vi "Red Pitaya Manager back.vi"() -> ()   [LabVIEW 2024]
uses:
  Libraries/Red Pitaya/RP Calibration.ctl
  Libraries/Red Pitaya/RP Calibration 4ch.ctl
  Libraries/Red Pitaya/RP Channel Calibration.ctl
  Libraries/Red Pitaya/RP Filter 4ch.ctl
  Libraries/Red Pitaya/RP Channel Filter.ctl
  Libraries/Red Pitaya/RP Calibration 2ch.ctl
  Libraries/Red Pitaya/RP Core/RP Communicator/RP Communicator.lvclass
  Libraries/Red Pitaya/RP Command.ctl
  Libraries/Red Pitaya/RP Config Offsets.ctl
  Libraries/Red Pitaya/RP Status Offsets.ctl
  <vilib>/regexp/Match Regular Expression.xnode
  Libraries/Red Pitaya/Red Pitaya Digitizer/Red Pitaya Digitizer.lvclass
panel:
  in  "Find Red Pitayas":bool
  out "Calibration":T1
  out "output cluster":T1
  in  "Tab Control":enum32{"Manage", "Settings", "Diagnostics"}(tab)
  in  "Frequencies":dbl[](array[numeric])=[0.0, 0.0]
  in  "Out enable":bool[](array[boolean])
  in  "Out gains":dbl[](array[numeric])=[1.0, 1.0]
  in  "Out offsets":i16[](array[numeric])=[0, 0]
  in  "Reset calibration":bool
  out "Waveform Chart":dbl[][](graph)
  in  "Input ranges":bool[](array[boolean])=[FALSE, FALSE, FALSE, FALSE]
  in  "In offsets":i32[](array[numeric])
  in  "In gains":dbl[](array[numeric])
  out "Calibrating":bool
  in  "Write callibration":bool
  in  "Stop calibration":bool
  in  "Start calibration":bool
  out "Starup script":string
  in  "View  startup":bool
  in  "View  bitfiles":bool
  in  "Red Pitayas":i32(listbox)
  out "bit files":string
  in  "bitfile functionality":string[](array[string])=["variable-rate digitizer", "lockin-digitizer", "slow lockin-digitizer", "lockin-digitizer  for 122.88", "fast 4-ch digitizer", "critical current", "slow critical current", "variable rate 4-ch digitizer"]
  in  "Bitfile logic tags 2":u16[](array[numeric])=[152, 159, 164, 169, 157, 154, 155, 158]
  in  "Subnet":string="192.168.1"
  in  "Start address":i32=100
  in  "End address":i32=120
  in  "Bitfile logic tags":u16[](array[numeric])=[101, 102, 109, 113, 159, 157, 152, 158]
  in  "Timeout":i32=100
  out "Bitfile IDs map":map{u16, string}(c390)={152="variable-rate digitizer", 154="critical current", 155="slow critical current", 157="fast 4-ch digitizer", 159="lockin-digitizer", 164="slow lockin-digitizer", 169="lockin-digitizer  for 122.88"}
  out "Addresses":string[](array[string])
  out "Device names":string[](array[string])
  out "Modules":i32[](array[numeric])
  out "DDS modula out":i64[](array[numeric])=[101, 102]
  out "Logic tags out":u16[](array[numeric])=[101, 102]
  in  "error in":errorcluster
  out "error out":errorcluster
  out "standard output":string
  out "standard error":string
  in  "Exit Button":bool
  # "typedef enum {\n    STEM_125_10_v1_0            = 0,\n    STEM_125_14_v1_0            = 1,\n    STEM_125_14_v1_1            = 2,\n    STEM_122_16SDR_v1_0         = 3,\n    STEM_122_16SDR_v1_1         = 4,\n    STEM_125_14_LN_v1_1         = 5,\n    STEM_125_14_Z7020_v1_0      = 6,\n    STEM_125_14_Z7020_LN_v1_1   = 7,\n    STEM_125_14_Z7020_4IN_v1_0  = 8,\n    STEM_125_14_Z7020_4IN_v1_2  = 9,\n    STEM_125_14_Z7020_4IN_v1_3  = 10,\n    STEM_250_12_v1_0            = 11,\n    STEM_250_12_v1_1            = 12,\n    STEM_250_12_v1_2            = 13,\n    STEM_250_12_120             = 14,\n    STEM_250_12_v1_2a           = 15,\n    STEM_250_12_v1_2b           = 16,\n    STEM_125_14_LN_BO_v1_1      = 17,\n    STEM_125_14_LN_CE1_v1_1     = 18,\n    STEM_125_14_LN_CE2_v1_1     = 19\n}  rp_HPeModels_t;"
  # "typedef enum {\n    Z7010 = 0,\n    Z7020 = 1\n}  rp_HPeZynqModels_t;"
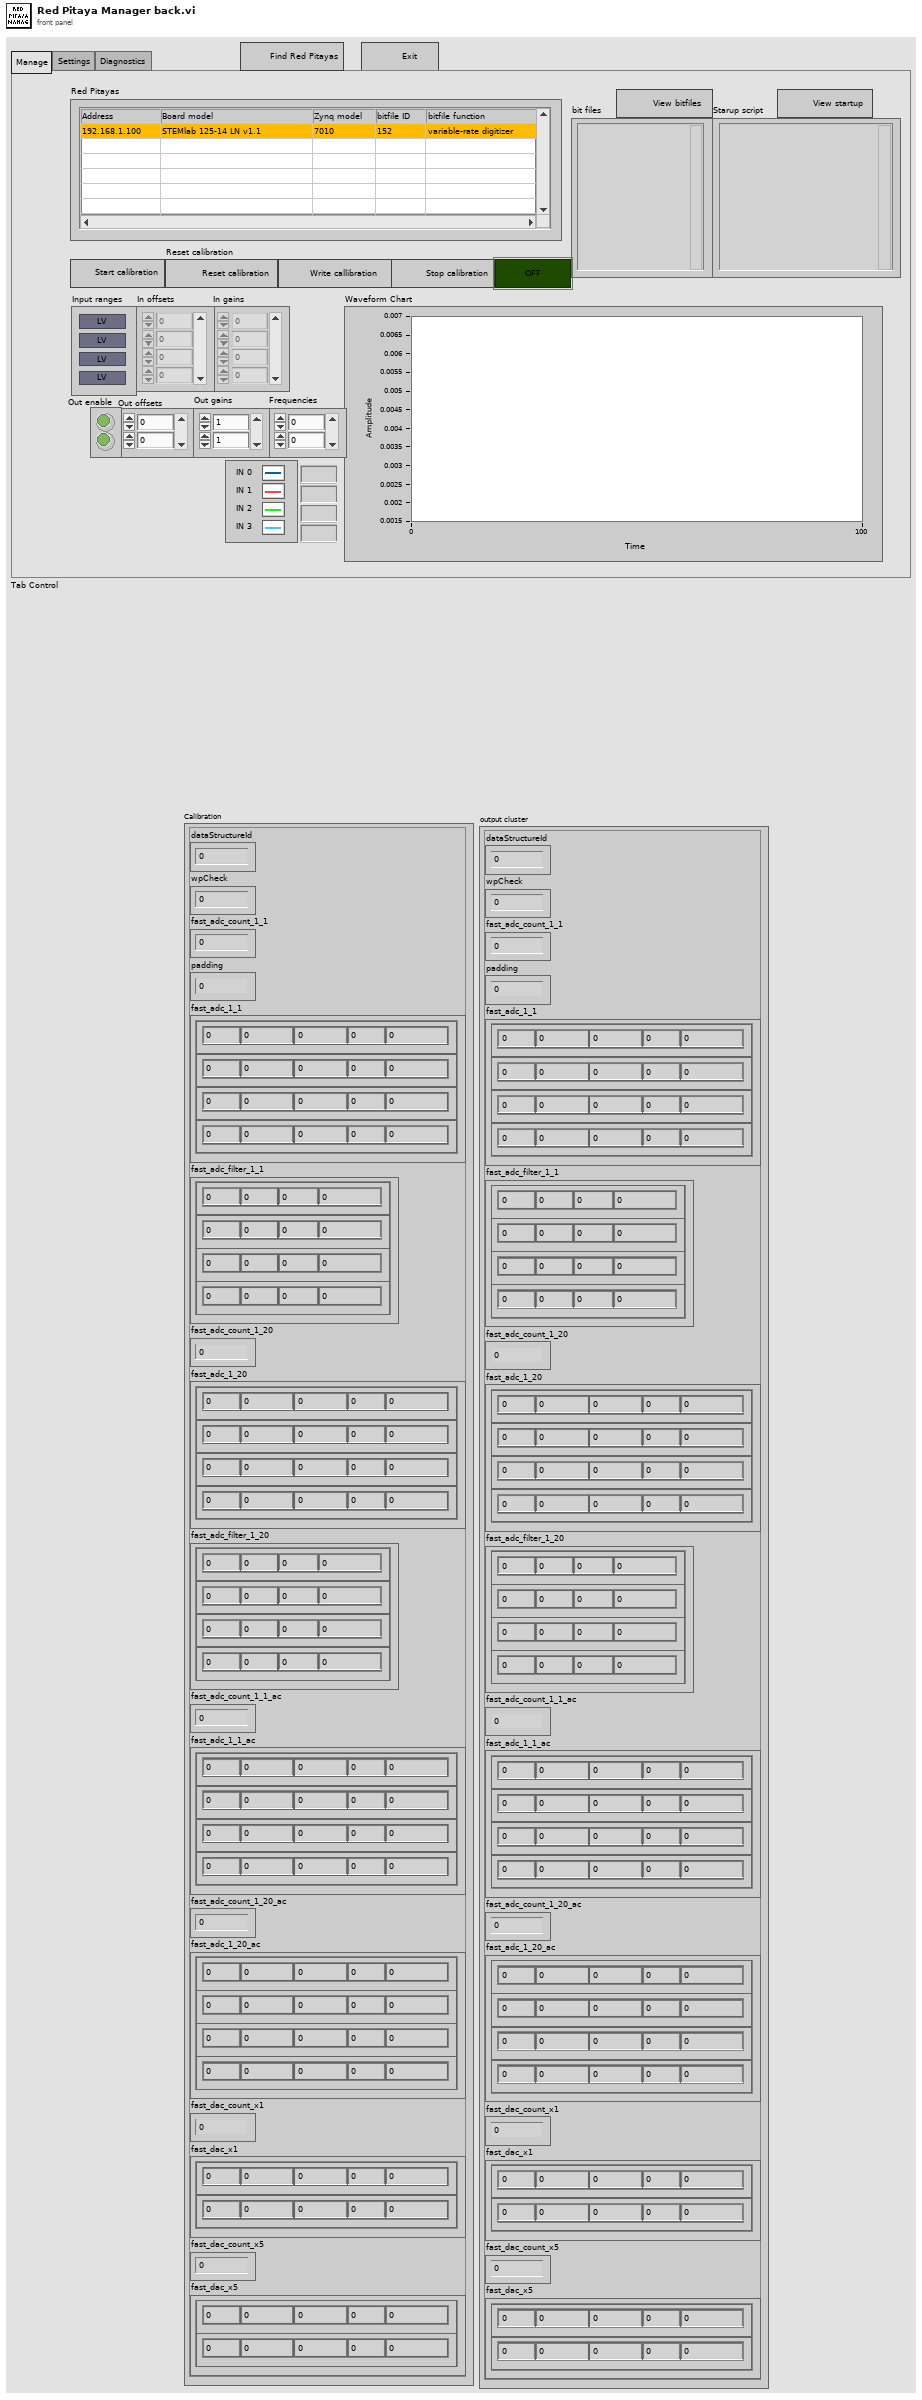
[diagram p1: front panel]
types:
  T1 = typedef "RP Calibration.ctl" = cluster{"dataStructureId":u8, "wpCheck":u8, "fast_adc_count_1_1":u16, "padding":u32, "fast_adc_1_1":T2, "fast_adc_filter_1_1":T4, "fast_adc_count_1_20":u64, "fast_adc_1_20":T2, "fast_adc_filter_1_20":T4, "fast_adc_count_1_1_ac":u64, "fast_adc_1_1_ac":T2, "fast_adc_count_1_20_ac":u64, "fast_adc_1_20_ac":T2, "fast_dac_count_x1":u64, "fast_dac_x1":T6, "fast_dac_count_x5":u64, "fast_dac_x5":T6}
  T2 = typedef "RP Calibration 4ch.ctl" = cluster{"ch_0":T3, "ch_1":T3, "ch_2":T3, "ch_3":T3}
  T3 = typedef "RP Channel Calibration.ctl" = cluster{"baseScale":sgl, "calibValue":u32, "offset":i32, "padding 2":i32, "gainCalc":dbl}
  T4 = typedef "RP Filter 4ch.ctl" = cluster{"ch_0":T5, "ch_1":T5, "ch_2":T5, "ch_3":T5}
  T5 = typedef "RP Channel Filter.ctl" = cluster{"aa":u32, "bb":u32, "pp":u32, "kk":u32}
  T6 = typedef "RP Calibration 2ch.ctl" = cluster{"ch_0":T3, "ch_1":T3}
  T7 = typedef "RP Command.ctl" = enum16{"Reset", "Read IDN", "Stop server", "Get status", "Get temperature", "Connect client", "Arm", "Software trigger", "Get whole buffer", "Get chunk", "System call", "Get config", "Set config", "Recieve data", "Recieve Calibartion", "Transmit data"}
  T8 = typedef "RP Config Offsets.ctl" = u16
  T9 = typedef "RP Status Offsets.ctl" = u16
  T10 = cluster{"fast_dac_x1[0]":T3, "fast_dac_x1[1]":T3}
  T11 = cluster{"fast_adc_1_1[0]":T3, "fast_adc_1_1[1]":T3, "fast_adc_1_1[2]":T3, "fast_adc_1_1[3]":T3}
  T12 = cluster{"fast_adc_1_20[0]":T3, "fast_adc_1_20[1]":T3, "fast_adc_1_20[2]":T3, "fast_adc_1_20[3]":T3}
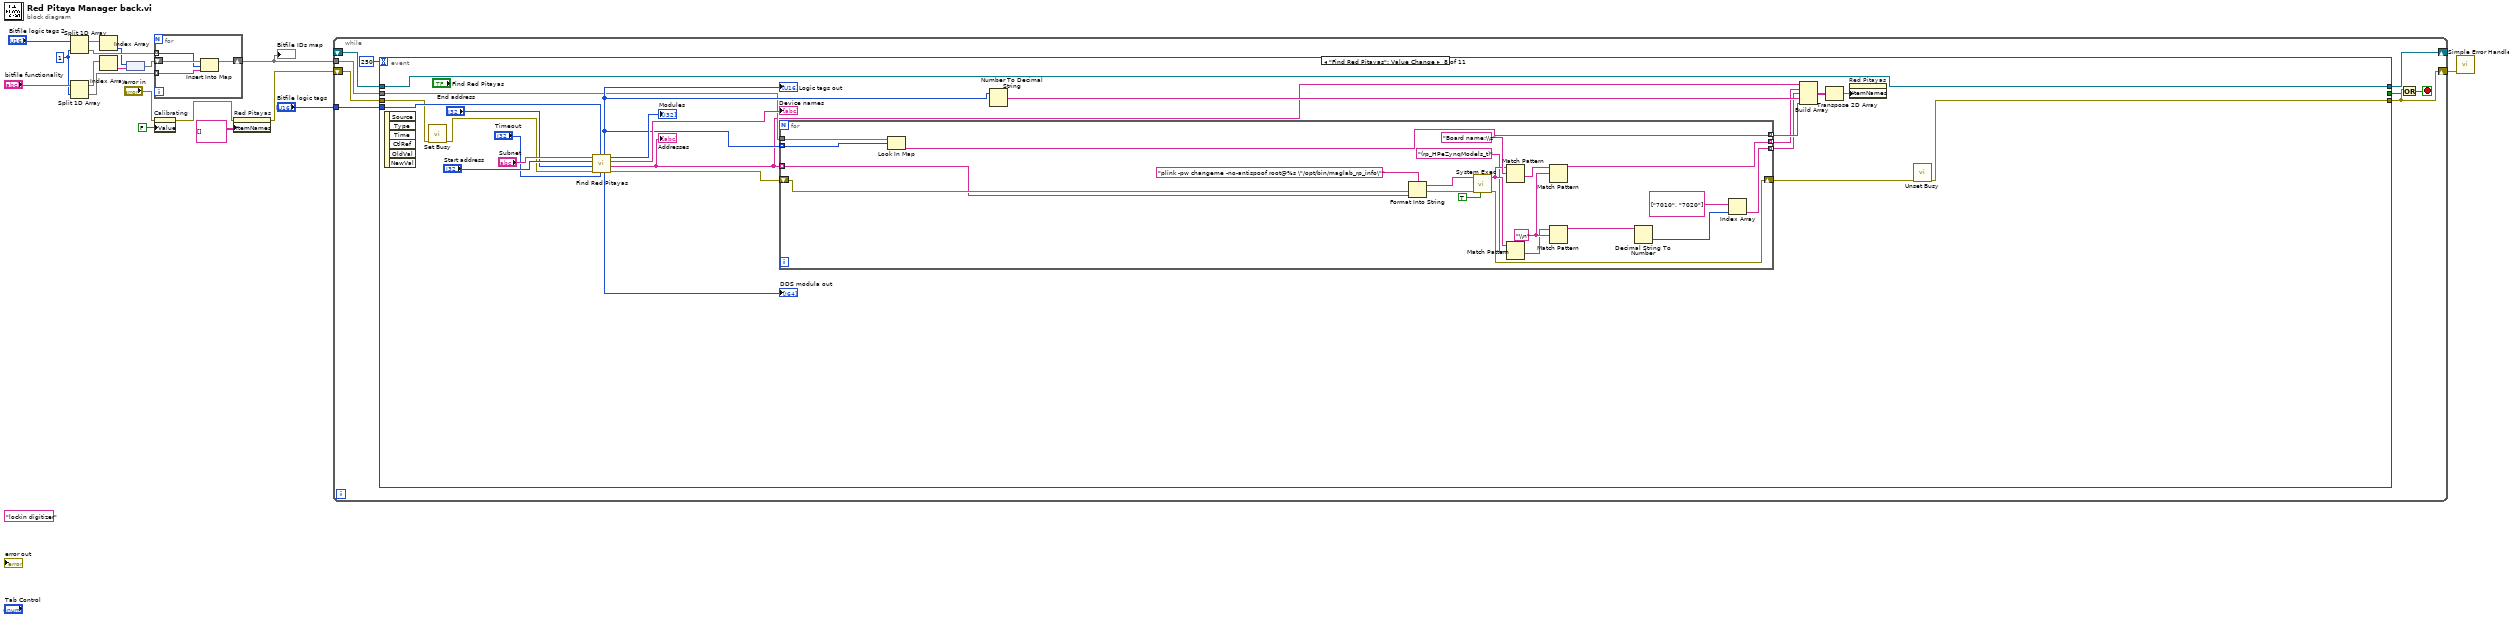
[diagram p0: block diagram]
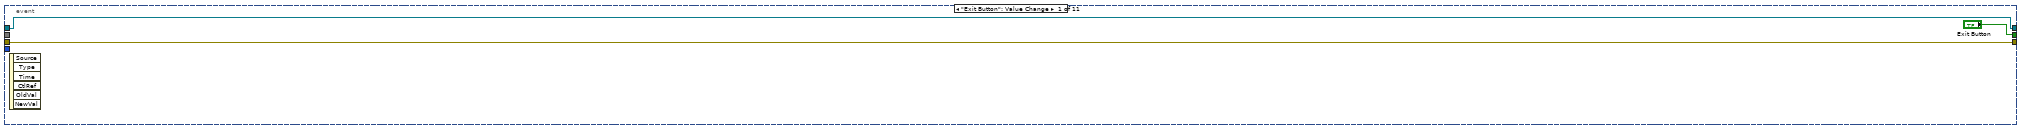
[diagram p2: hidden frame]
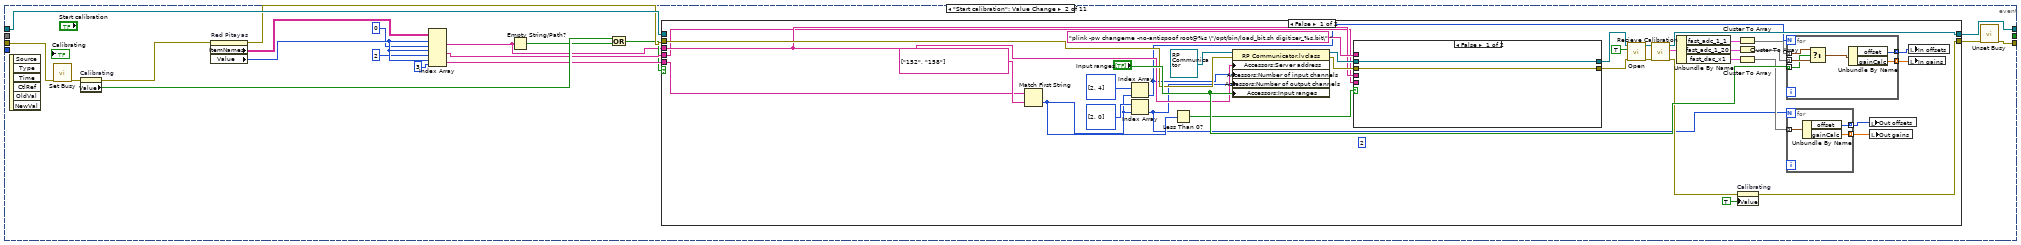
[diagram p3: hidden frame]
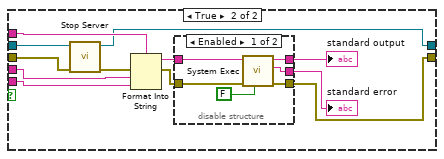
[diagram p4: hidden frame]
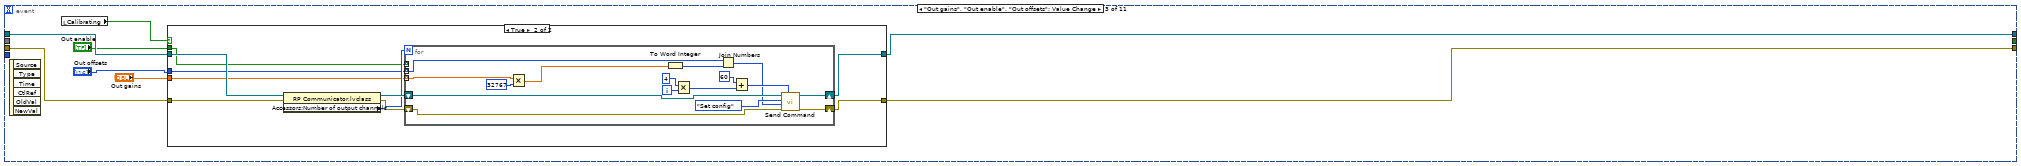
[diagram p7: hidden frame]
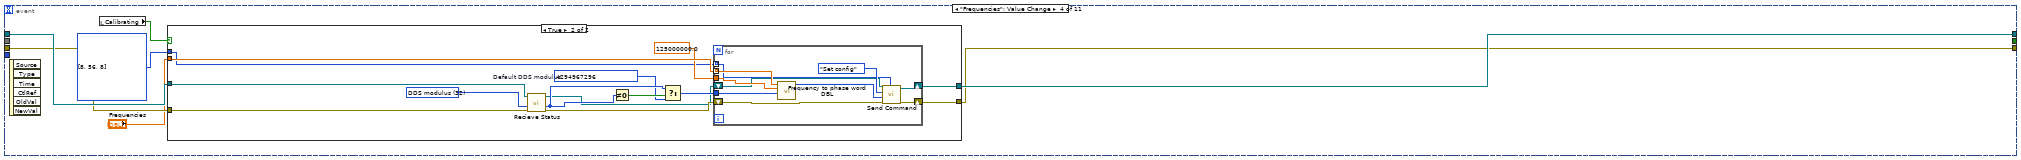
[diagram p9: hidden frame]
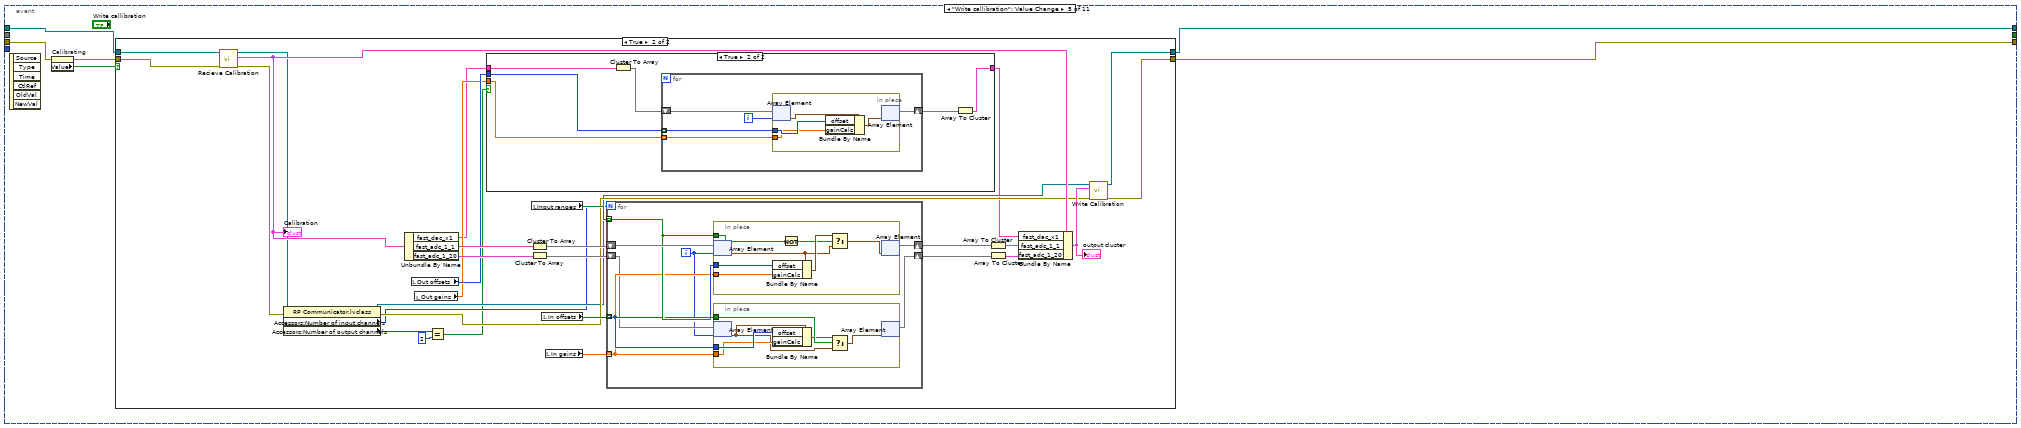
[diagram p11: hidden frame]
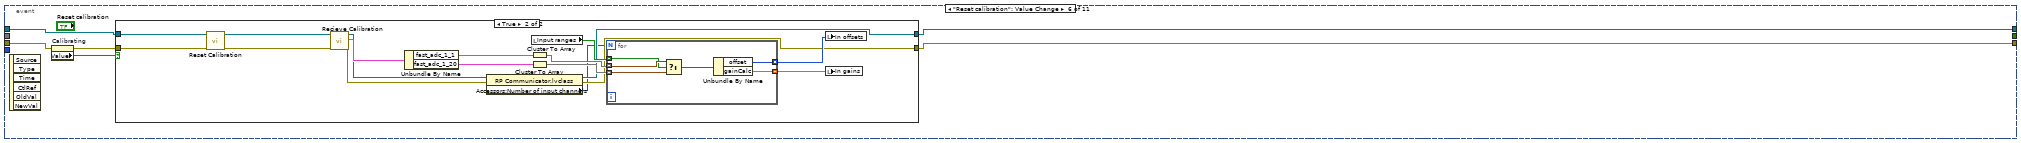
[diagram p14: hidden frame]
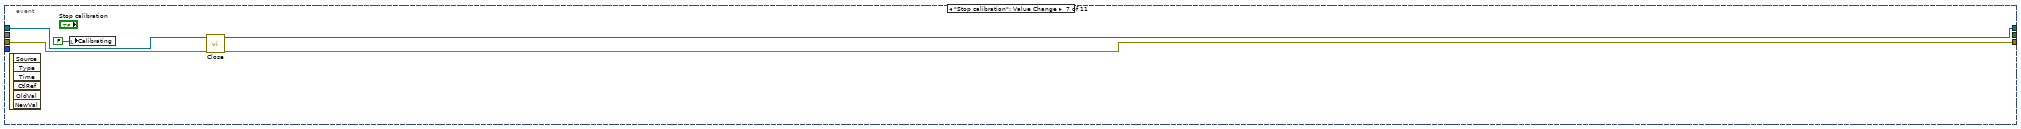
[diagram p16: hidden frame]
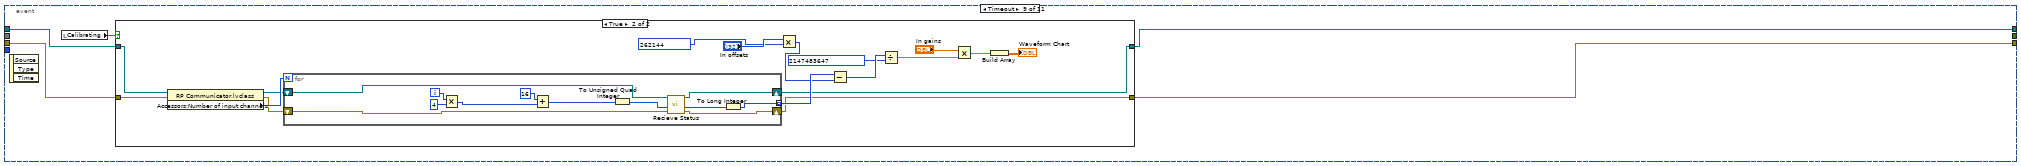
[diagram p17: hidden frame]
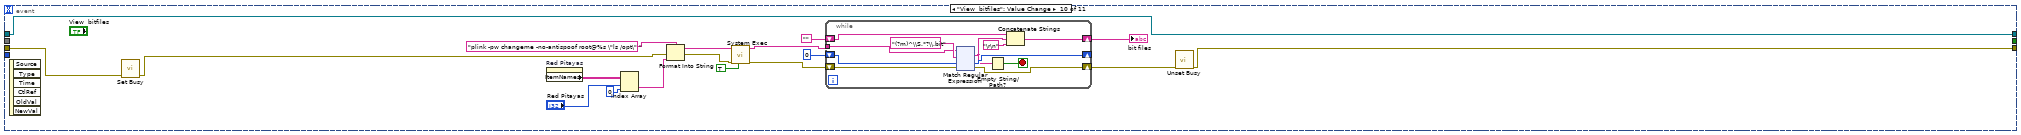
[diagram p19: hidden frame]
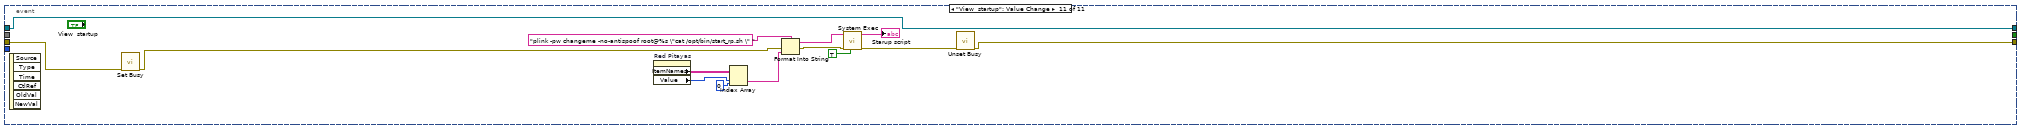
[diagram p20: hidden frame]
diagram:
  w15 = 1 ("index")
  (unwired) "lockin digitizer" ("value")
  n1 = Split 1D Array(array="Bitfile logic tags 2", index=w15) -> (first subarray=w14:u16[], second subarray=w12:u16[])
  n2 = Split 1D Array(array="bitfile functionality", index=w15) -> (first subarray=w13:string[], second subarray=w11:string[])
  n3 = Index Array(array=w14) -> (element=w9:u16)  [unwired: 1 in]
  n4 = Index Array(array=w13) -> (element=w8:string)  [unwired: 1 in]
  n5 = node(w9, w8) -> (w10:map{u16, string})
  n6 = for {
    tunnel: w12 -> [w21] mode=indexing
    tunnel: w11 -> [w20] mode=indexing
    shift-right: [w19] -> w7
    shift-left: w10 -> [w22]
    n7 = Insert Into Map(map in=w22, key=w21, value=w20) -> (map out=w19:map{u16, string})  [unwired: 2 out]
  }
  "Bitfile IDs map" <- w7
  n8 = property on="Calibrating" class="Bool (strict)"(error in="error in", "Value"=FALSE ("Calibrating")) -> (error out=w2:errorcluster)  [unwired: 1 in, 1 out]
  n9 = property on="Red Pitayas" class="MCListbox (strict)"(error in=w2, "ItemNames"=string[][] [] ("Item Names")) -> (error out=w1:errorcluster)  [unwired: 1 in, 1 out]
  n10 = while {
    tunnel: "Bitfile logic tags" -> [w31]
    tunnel: w7 -> [w30]
    shift-right: [w27] -> w6
    shift-left: w1 -> [w29]
    shift-right: [w24] -> _
    shift-left: _ -> [w23]
    stop <- w25 stop-if-true
    n11 = event shown="[7] \"Find Red Pitayas\": Value Change" {
      selector: _ -> [_ _ _ _ _ _ _ _ _ _ _]
      dyn-events: _ -> [_ _ _ _ _ _ _ _ _ _ _]
      timeout: 250 -> [_ _ _ _ _ _ _ _ _ _ _]
      tunnel: ["Exit Button" _ _ _ _ _ _ _ _ _ _] -> w26
      tunnel: w31 -> [_ _ _ _ _ _ _ w313 _ _ _]
      tunnel: w30 -> [_ _ _ _ _ _ _ w311 _ _ _]
      tunnel: w29 -> [w33 w51 w128 w160 w196 w270 w296 w305 w348 w391 w533]
      tunnel: [w33 w35 w127 w161 w192 w266 w297 w303 w347 w381 w527] -> w27
      tunnel: [w32 w52 w125 w162 w191 w265 w299 w301 w345 w385 w529] -> w24
      tunnel: w23 -> [w32 w49 w126 w163 w194 w267 w298 w301 w346 w385 w529]
      event "Exit Button": Value Change {
        n12 = event-data() -> ()  [unwired: 1 in, 6 out]
      }
      event "Start calibration": Value Change {
        n13 = event-data() -> ()  [unwired: 1 in, 6 out]
        n14 = call <vilib>:"Set Busy.vi"("error in (no error)"=w51) -> ("error out"=w36:errorcluster)  [unwired: 9 in, 1 out]
        n15 = property on="Calibrating" class="Bool (strict)"(error in=w36) -> (error out=w41:errorcluster, "Value"=w50:bool)  [unwired: 1 in, 1 out]
        n16 = property on="Red Pitayas" class="MCListbox (strict)"(error in=w41) -> (error out=w40:errorcluster, "ItemNames"=w47:string[][], "Value"=w48:i32)  [unwired: 1 in, 1 out]
        n17 = Index Array(array=w47, index (row) #1=w48, index (col) #1=0 ("disabled index (col)"), index (row) #2=w48, index (col) #2=2 ("disabled index (col)"), index (row) #3=w48, index (col) #3=3 ("disabled index (col)")) -> (element #1=w38:string, element #2=w43:string, element #3=w42:string)
        n18 = Empty String/Path?(string/path=w38) -> (empty?=w37:bool)
        n19 = Compound Arithmetic op=OR(w50, w37) -> (w39:bool)
        n20 = case shown="False" w39 {
          tunnel: [w75 w121] -> w53
          tunnel: [w85 w120] -> w52
          tunnel: w40 -> [w70 w121]
          tunnel: w49 -> [_ w120]
          tunnel: w38 -> [w65 _]
          tunnel: w43 -> [w64 _]
          tunnel: w42 -> [w63 _]
          frame False {
            (unwired) 2 ("Number of input channels")
            n21 = Match First String(2:string[] ["152", "158"] ("string array"), 3:w63) -> (0:w59:i32)  [unwired: 1 out]
            n22 = Index Array(array=i32[] [2, 4], index=w59) -> (element=w61:i32)
            n23 = Index Array(array=i32[] [2, 0], index=w59) -> (element=w56:i32)
            n24 = Less Than 0?(x=w59) -> (x < 0?=w66:bool)
            n25 = property class="RP Communicator.lvclass"(reference=refnum<class "RP Communicator.lvclass"> refnum ("RP Communicator.lvclass"), error in=w70, "Accessors:Server address"=w65, "Accessors:Number of input channels"=w61, "Accessors:Number of output channels"=w56, "Accessors:Input ranges"="Input ranges") -> (reference out=w73:refnum<class "RP Communicator.lvclass">, error out=w72:errorcluster)
            n26 = case shown="False" w66 {
              tunnel: "plink -pw changeme -no-antispoof root@%s \"/opt/bin/load_bit.sh digitizer_%s.bit\" " ("format string") -> [_ w104]
              tunnel: w64 -> [_ w101]
              tunnel: w65 -> [_ w100]
              tunnel: w73 -> [w93 w99]
              tunnel: w72 -> [w94 w98]
              tunnel: [w93 w97] -> w71
              tunnel: [w94 w95] -> w69
              frame False {
              }
              frame True {
                n27 = call-dynamic "Stop Server.vi"("error in (no error)"=w98, "RP Communicator in"=w99) -> ("error out"=w96:errorcluster, "RP Communicator out"=w97:refnum<class "RP Communicator.lvclass">)  [unwired: 8 in]
                n28 = Format Into String(format string=w104, error in=w96, w100, w101) -> (resulting string=w106:string, error out=w105:errorcluster)  [unwired: 1 in]
                n29 = disable-structure shown="Enabled" {
                  disable-tunnel: w106 -> [w112 _]
                  disable-tunnel: w105 -> [w111 w113]
                  disable-tunnel: [w110 _] -> w103
                  disable-tunnel: [w109 _] -> w102
                  disable-tunnel: [w108 w113] -> w95
                  frame Enabled {
                    n30 = call <vilib>:"System Exec.vi"("run minimized? (F)"=FALSE, "error in (no error)"=w111, "command line"=w112) -> ("error out"=w108:errorcluster, "standard error"=w109:string, "standard output"=w110:string)  [unwired: 5 in, 1 out]
                  }
                  frame Disabled {
                  }
                }
                "standard output" <- w103
                "standard error" <- w102
              }
            }
            n31 = call-dynamic "Open.vi"("error in (no error)"=w69, "Send \"Connect client\""=TRUE ("Send \"Connect client\""), "RP Communicator in"=w71) -> ("error out"=w87:errorcluster, "RP Communicator out"=w86:refnum<class "RP Communicator.lvclass">)  [unwired: 7 in]
            n32 = call-dynamic "Recieve Calibration.vi"("error in (no error)"=w87, "RP Communicator in"=w86) -> ("error out"=w76:errorcluster, "Calibration"=w84:T1, "RP Communicator out"=w85:refnum<class "RP Communicator.lvclass">)  [unwired: 7 in]
            n33 = Unbundle By Name(w84) -> ("fast_adc_1_1"=w83:T2, "fast_adc_1_20"=w82:T2, "fast_dac_x1"=w58:T6)
            n34 = property on="Calibrating" class="Bool (strict)"(error in=w76, "Value"=TRUE ("Calibrating")) -> (error out=w75:errorcluster)  [unwired: 1 in, 1 out]
            n35 = Cluster To Array(cluster=w83) -> (array=w81:T3[])
            n36 = Cluster To Array(cluster=w82) -> (array=w80:T3[])
            n37 = Cluster To Array(cluster=w58) -> (array=w57:T3[])
            n38 = for {
              N: w61 -> [_]
              tunnel: w81 -> [w119] mode=indexing
              tunnel: w80 -> [w118] mode=indexing
              tunnel: "Input ranges" -> [w117] mode=indexing
              tunnel: [w115] -> w77 mode=indexing
              tunnel: [w114] -> w78 mode=indexing
              n39 = Select(t=w119, s=w117, f=w118) -> (s? t:f=w116:T3)
              n40 = Unbundle By Name(w116) -> ("offset"=w114:i32, "gainCalc"=w115:dbl)
            }
            n41 = for {
              N: w56 -> [_]
              tunnel: w57 -> [w92] mode=indexing
              tunnel: [w91] -> w54 mode=indexing
              tunnel: [w90] -> w55 mode=indexing
              n42 = Unbundle By Name(w92) -> ("offset"=w91:i32, "gainCalc"=w90:dbl)
            }
            n43 = local write "Out offsets"(w54) -> ()
            n44 = local write "Out gains"(w55) -> ()
            n45 = local write "In offsets"(w78) -> ()
            n46 = local write "In gains"(w77) -> ()
          }
          frame True {
          }
        }
        n47 = call <vilib>:"Unset Busy.vi"("error in (no error)"=w53) -> ("error out"=w35:errorcluster)  [unwired: 10 in]
      }
      event "Out gains", "Out enable", "Out offsets": Value Change {
        n48 = event-data() -> ()  [unwired: 1 in, 6 out]
        n49 = local read "Calibrating"() -> (w129:bool)
        n50 = case shown="True" w129 {
          tunnel: w128 -> [w131 w137]
          tunnel: [w131 w135] -> w127
          tunnel: w126 -> [w130 w141]
          tunnel: [w130 w140] -> w125
          tunnel: "Out offsets" -> [_ w134]
          tunnel: "Out enable" -> [_ w133]
          tunnel: "Out gains" -> [_ w132]
          frame False {
          }
          frame True {
            n51 = property class="RP Communicator.lvclass"(reference=w141, error in=w137) -> (reference out=w139:refnum<class "RP Communicator.lvclass">, error out=w136:errorcluster, "Accessors:Number of output channels"=w138:i32)
            n52 = for {
              N: w138 -> [_]
              tunnel: w133 -> [_] mode=indexing
              tunnel: w134 -> [w144] mode=indexing
              tunnel: w132 -> [w147] mode=indexing
              shift-right: [w156] -> w140
              shift-left: w139 -> [w157]
              shift-right: [w148] -> w135
              shift-left: w136 -> [w149]
              i -> [w152]
              n53 = Multiply(x=w147, y=i16 32767) -> (x*y=w146:dbl)
              n54 = To Word Integer(number=w146) -> (16bit integer=w145:i16)
              n55 = Multiply(x=4, y=w152) -> (x*y=w151:i32)
              n56 = Join Numbers(hi=w144, lo=w145) -> ((hi.lo)=w143:u32)
              n57 = Add(x=60, y=w151) -> (x+y=w150:i32)
              n58 = call-dynamic "Send Command.vi"("Config offset"=w150, "error in (no error)"=w149, "Command payload"=w143, "Command number"=RP_Command."Set config", "RP Communicator in"=w157) -> ("error out"=w148:errorcluster, "RP Communicator out"=w156:refnum<class "RP Communicator.lvclass">)  [unwired: 4 in, 1 out]
            }
          }
        }
      }
      event "Frequencies": Value Change {
        w158 = T8[] [8, 56, 8] items=["Config flags"=0, "Record length"=4, "Frequency 0"=8, "Decimation"=12, "LED"=16, "DDS delay"=28, "Fequency 1"=56]
        n59 = event-data() -> ()  [unwired: 1 in, 6 out]
        n60 = local read "Calibrating"() -> (w164:bool)
        n61 = case shown="True" w164 {
          tunnel: w163 -> [w166 w178]
          tunnel: [w166 w169] -> w162
          tunnel: [w165 w168] -> w161
          tunnel: w160 -> [w165 w177]
          tunnel: "Frequencies" -> [_ w180]
          tunnel: w158 -> [_ w167]
          frame False {
          }
          frame True {
            w173 = i64 4294967296  # Default DDS modulus
            w176 = T9 32 items=["Writer address"=0, "Record start position"=4, "Trig state and ID"=8, "Phase"=12, "X1"=16, "Y1"=20, "RxFIFO counter or  X2"=24, "TxFIFO counter or Y2"=28, "DDS modulus"=32] ("Status offsets")
            n62 = call-dynamic "Recieve Status.vi"("error in (no error)"=w177, "Status offset"=w176, "RP Communicator in"=w178) -> ("error out"=w171:errorcluster, "Status response"=w174:u32, "RP Communicator out"=w170:refnum<class "RP Communicator.lvclass">)  [unwired: 6 in]
            n63 = Not Equal To 0?(x=w174) -> (x != 0?=w175:bool)
            n64 = Select(t=w174, s=w175, f=w173) -> (s? t:f=w172:i64)
            n65 = for {
              tunnel: w180 -> [w190] mode=indexing
              tunnel: 125000000.0 ("DDS clock") -> [w189]
              tunnel: w172 -> [w188]
              shift-right: [w183] -> w168
              shift-left: w171 -> [w187]
              shift-right: [w184] -> w169
              shift-left: w170 -> [w185]
              tunnel: w167 -> [w182] mode=indexing
              n66 = call "Frequency to phase word DBL.vi"("DDS modulus"=w188, "DDS clock"=w189, "Frequency"=w190) -> ("Phase word"=w181:u64)  [unwired: 7 in, 1 out]
              n67 = call-dynamic "Send Command.vi"("Config offset"=w182, "error in (no error)"=w187, "Command payload"=w181, "Command number"=RP_Command."Set config", "RP Communicator in"=w185) -> ("error out"=w183:errorcluster, "RP Communicator out"=w184:refnum<class "RP Communicator.lvclass">)  [unwired: 4 in, 1 out]
            }
          }
        }
      }
      event "Write callibration": Value Change {
        n68 = event-data() -> ()  [unwired: 1 in, 6 out]
        n69 = property on="Calibrating" class="Bool (strict)"(error in=w196) -> (error out=w193:errorcluster, "Value"=w195:bool)  [unwired: 1 in, 1 out]
        n70 = case shown="True" w195 {
          tunnel: w194 -> [w198 w227]
          tunnel: w193 -> [w197 w226]
          tunnel: [w197 w211] -> w192
          tunnel: [w198 w213] -> w191
          frame False {
          }
          frame True {
            n71 = call-dynamic "Recieve Calibration.vi"("error in (no error)"=w226, "RP Communicator in"=w227) -> ("error out"=w212:errorcluster, "Calibration"=w217:T1, "RP Communicator out"=w208:refnum<class "RP Communicator.lvclass">)  [unwired: 7 in]
            "Calibration" <- w217
            n72 = property class="RP Communicator.lvclass"(reference=w208, error in=w212) -> (reference out=w207:refnum<class "RP Communicator.lvclass">, error out=w209:errorcluster, "Accessors:Number of input channels"=w206:i32, "Accessors:Number of output channels"=w203:i32)
            n73 = Unbundle By Name(w217) -> ("fast_dac_x1"=w199:T6, "fast_adc_1_1"=w222:T2, "fast_adc_1_20"=w221:T2)
            n74 = local read "Out offsets"() -> (w205:i16[])
            n75 = local read "Out gains"() -> (w204:dbl[])
            n76 = Equal?(x=w203, y=2) -> (x = y?=w201:bool)
            n77 = case shown="True" w201 {
              tunnel: w199 -> [w228 w234]
              tunnel: w205 -> [_ w232]
              tunnel: w204 -> [_ w231]
              tunnel: [w228 w229] -> w200
              frame False {
              }
              frame True {
                n78 = Cluster To Array(cluster=w234) -> (array=w233:T3[])
                n79 = for {
                  tunnel: w232 -> [w239] mode=indexing
                  tunnel: w231 -> [w238] mode=indexing
                  shift-right: [w235] -> w230
                  shift-left: w233 -> [w237]
                  i -> [w236]
                  n80 = in-place {
                    in-place-border: w239 -> [w243]
                    in-place-border: w238 -> [w242]
                    n81 = in-place-array #1(w237, w236) -> (w241:T3)
                    n82 = Bundle By Name(cluster=w241, "offset"=w243, "gainCalc"=w242) -> (w240:T3)
                    n83 = in-place-array #1(w240) -> (w235:T3[])  [unwired: 1 out]
                  }
                }
                n84 = Array To Cluster(array=w230) -> (cluster=w229:T10)
              }
            }
            n85 = Cluster To Array(cluster=w222) -> (array=w220:T3[])
            n86 = Cluster To Array(cluster=w221) -> (array=w219:T3[])
            n87 = local read "Input ranges"() -> (w225:bool[])
            n88 = local read "In offsets"() -> (w224:i32[])
            n89 = local read "In gains"() -> (w223:dbl[])
            n90 = for {
              N: w206 -> [_]
              tunnel: w225 -> [w250] mode=indexing
              tunnel: w224 -> [w249] mode=indexing
              tunnel: w223 -> [w248] mode=indexing
              shift-right: [w245] -> w218
              shift-left: w220 -> [w251]
              shift-right: [w244] -> w215
              shift-left: w219 -> [w247]
              i -> [w246]
              n91 = in-place {
                in-place-border: w250 -> [w257]
                in-place-border: w249 -> [w256]
                in-place-border: w248 -> [w255]
                n92 = in-place-array #2(w251, w246) -> (w253:T3)
                n93 = Bundle By Name(cluster=w253, "offset"=w256, "gainCalc"=w255) -> (w258:T3)
                n94 = Not(x=w257) -> (.not. x?=w252:bool)
                n95 = Select(t=w258, s=w252, f=w253) -> (s? t:f=w254:T3)
                n96 = in-place-array #2(w254) -> (w245:T3[])  [unwired: 1 out]
              }
              n97 = in-place {
                in-place-border: w250 -> [w264]
                in-place-border: w249 -> [w263]
                in-place-border: w248 -> [w262]
                n98 = in-place-array #3(w247, w246) -> (w260:T3)
                n99 = Bundle By Name(cluster=w260, "offset"=w263, "gainCalc"=w262) -> (w259:T3)
                n100 = Select(t=w259, s=w264, f=w260) -> (s? t:f=w261:T3)
                n101 = in-place-array #3(w261) -> (w244:T3[])  [unwired: 1 out]
              }
            }
            n102 = Array To Cluster(array=w218) -> (cluster=w216:T11)
            n103 = Array To Cluster(array=w215) -> (cluster=w214:T12)
            n104 = Bundle By Name(cluster=w217, "fast_dac_x1"=w200, "fast_adc_1_1"=w216, "fast_adc_1_20"=w214) -> (w210:T1)
            "output cluster" <- w210
            n105 = call-dynamic "Write Calibration.vi"("error in (no error)"=w209, "Calibration"=w210, "RP Communicator in"=w207) -> ("error out"=w211:errorcluster, "RP Communicator out"=w213:refnum<class "RP Communicator.lvclass">)  [unwired: 7 in]
          }
        }
      }
      event "Reset calibration": Value Change {
        n106 = event-data() -> ()  [unwired: 1 in, 6 out]
        n107 = property on="Calibrating" class="Bool (strict)"(error in=w270) -> (error out=w268:errorcluster, "Value"=w269:bool)  [unwired: 1 in, 1 out]
        n108 = case shown="True" w269 {
          tunnel: w268 -> [w272 w289]
          tunnel: w267 -> [w271 w288]
          tunnel: [w272 w276] -> w266
          tunnel: [w271 w274] -> w265
          frame False {
          }
          frame True {
            n109 = call-dynamic "Reset Calibration.vi"("error in (no error)"=w289, "RP Communicator in"=w288) -> ("error out"=w282:errorcluster, "RP Communicator out"=w281:refnum<class "RP Communicator.lvclass">)  [unwired: 8 in]
            n110 = call-dynamic "Recieve Calibration.vi"("error in (no error)"=w282, "RP Communicator in"=w281) -> ("error out"=w278:errorcluster, "Calibration"=w287:T1, "RP Communicator out"=w275:refnum<class "RP Communicator.lvclass">)  [unwired: 7 in]
            n111 = Unbundle By Name(w287) -> ("fast_adc_1_1"=w286:T2, "fast_adc_1_20"=w285:T2)
            n112 = property class="RP Communicator.lvclass"(reference=w275, error in=w278) -> (reference out=w274:refnum<class "RP Communicator.lvclass">, error out=w276:errorcluster, "Accessors:Number of input channels"=w273:i32)
            n113 = Cluster To Array(cluster=w286) -> (array=w284:T3[])
            n114 = Cluster To Array(cluster=w285) -> (array=w283:T3[])
            n115 = local read "Input ranges"() -> (w280:bool[])
            n116 = for {
              N: w273 -> [_]
              tunnel: w284 -> [w295] mode=indexing
              tunnel: w283 -> [w294] mode=indexing
              tunnel: w280 -> [w293] mode=indexing
              tunnel: [w291] -> w277 mode=indexing
              tunnel: [w290] -> w279 mode=indexing
              n117 = Select(t=w295, s=w293, f=w294) -> (s? t:f=w292:T3)
              n118 = Unbundle By Name(w292) -> ("offset"=w290:i32, "gainCalc"=w291:dbl)
            }
            n119 = local write "In offsets"(w279) -> ()
            n120 = local write "In gains"(w277) -> ()
          }
        }
      }
      event "Stop calibration": Value Change {
        n121 = event-data() -> ()  [unwired: 1 in, 6 out]
        n122 = local write "Calibrating"(FALSE ("Calibrating")) -> ()
        n123 = call-dynamic "Close.vi"("error in (no error)"=w296, "RP Communicator in"=w298) -> ("error out"=w297:errorcluster, "RP Communicator out"=w299:refnum<class "RP Communicator.lvclass">)  [unwired: 8 in]
      }
      event "Find Red Pitayas": Value Change {
        n124 = event-data() -> ()  [unwired: 1 in, 6 out]
        n125 = call <vilib>:"Set Busy.vi"("error in (no error)"=w305) -> ("error out"=w304:errorcluster)  [unwired: 9 in, 1 out]
        n126 = call "Find Red Pitayas.vi"("Timeout"="Timeout", "Acceptable logic tags"=w313, "Error In"=w304, "End address"="End address", "Start address"="Start address", "Subnet"="Subnet") -> ("Error Out"=w309:errorcluster, "Addresses"=w308:string[], "Device names"=→"Device names":string[], "Modules"=→"Modules":i32[], "DDS modula out"=→"DDS modula out":i64[], "Logic tags out"=w312:u16[])
        "Logic tags out" <- w312
        "Addresses" <- w308
        n127 = for {
          tunnel: w312 -> [w343] mode=indexing
          tunnel: w311 -> [w344]
          tunnel: [w342] -> w310 mode=indexing
          shift-right: [w336] -> w302
          shift-left: w309 -> [w338]
          tunnel: w308 -> [w335] mode=indexing
          tunnel: [w332] -> w307 mode=indexing
          tunnel: [w325] -> w306 mode=indexing
          w329 = "\\n"
          n128 = Look In Map(map=w344, key=w343) -> (value=w342:string)  [unwired: 1 in, 1 out]
          n129 = Format Into String(format string="plink -pw changeme -no-antispoof root@%s \"/opt/bin/maglab_rp_info\"", error in=w338, w335) -> (resulting string=w340:string, error out=w337:errorcluster)  [unwired: 1 in]
          n130 = call <vilib>:"System Exec.vi"("run minimized? (F)"=TRUE, "error in (no error)"=w337, "command line"=w340) -> ("error out"=w336:errorcluster, "standard output"=w331:string)  [unwired: 5 in, 2 out]
          n131 = Match Pattern(string=w331, regular expression="Board name:\\s") -> (after substring=w333:string)  [unwired: 1 in, 3 out]
          n132 = Match Pattern(string=w331, regular expression="(rp_HPeZynqModels_t)") -> (after substring=w328:string)  [unwired: 1 in, 3 out]
          n133 = Match Pattern(string=w333, regular expression=w329) -> (before substring=w332:string)  [unwired: 1 in, 3 out]
          n134 = Match Pattern(string=w328, regular expression=w329) -> (before substring=w324:string)  [unwired: 1 in, 3 out]
          n135 = Decimal String To Number(string=w324) -> (number=w327:i32)  [unwired: 2 in, 1 out]
          n136 = Index Array(array=string[] ["7010", "7020"], index=w327) -> (element=w325:string)
        }
        n137 = Number To Decimal String(number=w312) -> (decimal integer string=w316:string[])  [unwired: 1 in]
        n138 = Build Array(w308, w307, w306, w316, w310) -> (w315:string[][])
        n139 = Transpose 2D Array(2D array=w315) -> (transposed array=w314:string[][])
        n140 = property on="Red Pitayas" class="MCListbox (strict)"("ItemNames"=w314) -> ()  [unwired: 2 in, 2 out]
        n141 = call <vilib>:"Unset Busy.vi"("error in (no error)"=w302) -> ("error out"=w303:errorcluster)  [unwired: 10 in]
      }
      event Timeout {
        n142 = event-data() -> ()  [unwired: 1 in, 3 out]
        n143 = local read "Calibrating"() -> (w349:bool)
        n144 = case shown="True" w349 {
          tunnel: w348 -> [w351 w364]
          tunnel: [w351 w356] -> w347
          tunnel: w346 -> [w350 w368]
          tunnel: [w350 w357] -> w345
          frame False {
          }
          frame True {
            n145 = property class="RP Communicator.lvclass"(reference=w368, error in=w364) -> (reference out=w366:refnum<class "RP Communicator.lvclass">, error out=w365:errorcluster, "Accessors:Number of input channels"=w367:i32)
            n146 = for {
              N: w367 -> [_]
              shift-right: [w379] -> w357
              shift-left: w366 -> [w380]
              shift-right: [w371] -> w356
              shift-left: w365 -> [w372]
              tunnel: [w369] -> w363 mode=indexing
              i -> [w378]
              n147 = Multiply(x=w378, y=4) -> (x*y=w375:i32)
              n148 = Add(x=16, y=w375) -> (x+y=w374:i32)
              n149 = To Unsigned Quad Integer(1:w374) -> (0:w373:u64)
              n150 = call-dynamic "Recieve Status.vi"("error in (no error)"=w372, "Status offset"=w373, "RP Communicator in"=w380) -> ("error out"=w371:errorcluster, "Status response"=w370:u32, "RP Communicator out"=w379:refnum<class "RP Communicator.lvclass">)  [unwired: 6 in]
              n151 = To Long Integer(number=w370) -> (32bit integer=w369:i32)
            }
            n152 = Multiply(x="In offsets", y=262144) -> (x*y=w354:i32[])
            n153 = Subtract(x=w363, y=w354) -> (x-y=w362:i32[])
            n154 = Divide(x=w362, y=2147483647) -> (x/y=w360:dbl[])
            n155 = Multiply(x="In gains", y=w360) -> (x*y=w358:dbl[])
            n156 = Build Array(w358) -> (→"Waveform Chart":dbl[][])
          }
        }
      }
      event "View  bitfiles": Value Change {
        n157 = event-data() -> ()  [unwired: 1 in, 6 out]
        n158 = call <vilib>:"Set Busy.vi"("error in (no error)"=w391) -> ("error out"=w382:errorcluster)  [unwired: 9 in, 1 out]
        n159 = property on="Red Pitayas" class="MCListbox (strict)"() -> ("ItemNames"=w394:string[][])  [unwired: 2 in, 2 out]
        n160 = Index Array(array=w394, index (row)="Red Pitayas", index (col)=0 ("disabled index (col)")) -> (element=w390:string)
        n161 = Format Into String(format string="plink -pw changeme -no-antispoof root@%s \"ls /opt\" ", error in=w382, w390) -> (resulting string=w397:string, error out=w395:errorcluster)  [unwired: 1 in]
        n162 = call <vilib>:"System Exec.vi"("run minimized? (F)"=TRUE, "error in (no error)"=w395, "command line"=w397) -> ("error out"=w383:errorcluster, "standard output"=w386:string)  [unwired: 5 in, 2 out]
        n163 = while {
          shift-right: [w402] -> w387
          shift-left: "" -> [w408]
          shift-right: [w406] -> w384
          shift-left: w383 -> [w405]
          shift-right: [w404] -> _
          shift-left: 0 ("offset past match") -> [w403]
          tunnel: w386 -> [w399]
          stop <- w400 stop-if-true
          n164 = xnode "Match Regular Expression"("input string"=w399, "regular expression"="(?m)^\\S.*?\\.bit", "offset (0)"=w403, "error in"=w405) -> ("whole match"=w401:string, "offset past match"=w404:i32, "error out"=w406:errorcluster)  [unwired: 2 in, 2 out]
          n165 = Empty String/Path?(string/path=w401) -> (empty?=w400:bool)
          n166 = Concatenate Strings(w408, w401, "\r\n") -> (w402:string)
        }
        "bit files" <- w387
        n167 = call <vilib>:"Unset Busy.vi"("error in (no error)"=w384) -> ("error out"=w381:errorcluster)  [unwired: 10 in]
      }
      event "View  startup": Value Change {
        n168 = event-data() -> ()  [unwired: 1 in, 6 out]
        n169 = call <vilib>:"Set Busy.vi"("error in (no error)"=w533) -> ("error out"=w528:errorcluster)  [unwired: 9 in, 1 out]
        n170 = property on="Red Pitayas" class="MCListbox (strict)"() -> ("ItemNames"=w534:string[][], "Value"=w532:i32)  [unwired: 2 in, 2 out]
        n171 = Index Array(array=w534, index (row)=w532, index (col)=0 ("disabled index (col)")) -> (element=w535:string)
        n172 = Format Into String(format string="plink -pw changeme -no-antispoof root@%s \"cat /opt/bin/start_rp.sh \" ", error in=w528, w535) -> (resulting string=w539:string, error out=w537:errorcluster)  [unwired: 1 in]
        n173 = call <vilib>:"System Exec.vi"("run minimized? (F)"=TRUE, "error in (no error)"=w537, "command line"=w539) -> ("error out"=w530:errorcluster, "standard output"=→"Starup script":string)  [unwired: 5 in, 2 out]
        n174 = call <vilib>:"Unset Busy.vi"("error in (no error)"=w530) -> ("error out"=w527:errorcluster)  [unwired: 10 in]
      }
    }
    n175 = Or(x=w27, y=w26) -> (x .or. y?=w25:bool)
  }
  n176 = call <vilib>:"Simple Error Handler.vi"("error in (no error)"=w6) -> ()  [unwired: 4 in, 5 out]
